vi "getAndorErrorCode.vi"(8 "error in (no error)":errorcluster, 11 "AndorController.lvclass in":refnum<class "AndorController.lvclass">) -> (0 "error out":errorcluster, 2 "Andor Error Codes":dbl[](array[numeric]), 3 "AndorController.lvclass out":refnum<class "AndorController.lvclass">)   [LabVIEW 2009, in "Hardware.lvlib" / "Channels.lvlib" / "AndorController.lvclass"]
uses:
  AndorController.lvclass
  AndorController.lvclass/AndorController.ctl
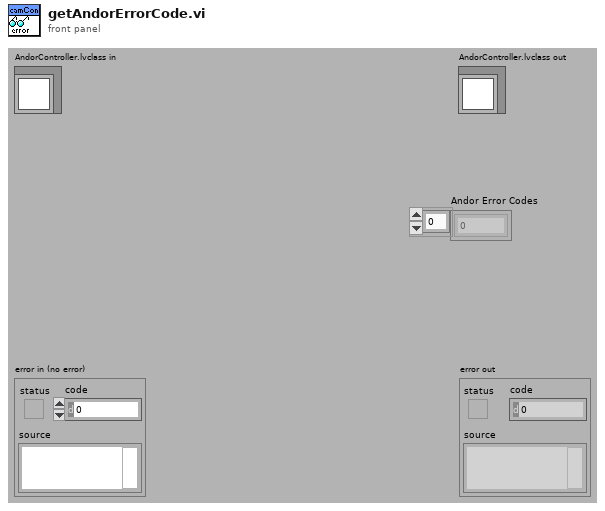
[diagram p1: front panel]
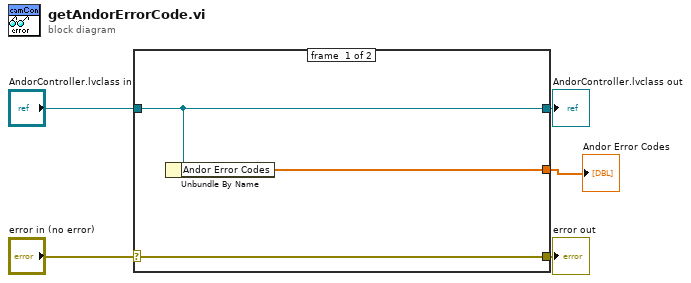
[diagram p0: block diagram]
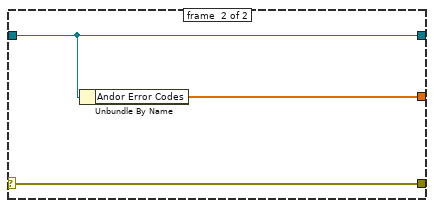
[diagram p2: hidden frame]
diagram:
  n1 = case shown="No Error" "error in (no error)" {
    selector: "error in (no error)" -> [w8 w11]
    tunnel: [w8 w11] -> w4
    tunnel: [w7 w10] -> w2
    tunnel: "AndorController.lvclass in" -> [w7 w10]
    tunnel: [w6 w9] -> w1
    frame #0 {
      n2 = Unbundle By Name(w7) -> ("Andor Error Codes"=w6:dbl[])
    }
    frame #1 {
      n3 = Unbundle By Name(w10) -> ("Andor Error Codes"=w9:dbl[])
    }
  }
  "error out" <- w4
  "AndorController.lvclass out" <- w2
  "Andor Error Codes" <- w1
